vi "超标留样启动流程.vi"   [LabVIEW 2016, in "超标留样集成.lvlib" / "德润DR803M超标留样.lvlib"]
types:
  T1 = cluster{"仪器时间":timestamp, "工作状态":u16, "工作进程":u16, "采样模式":u16, "采样瓶数":dbl, "当前瓶号":dbl, "设定平行样数":dbl, "已采平行样":dbl, "设定每瓶采样次数":dbl, "已采次数":dbl, "当前瓶采样量":dbl, "瞬时流量":dbl, "累积流量":dbl, "混匀桶已采次数":dbl, "COD":dbl, "NH3N":dbl, "门状态":u16, "采样泵使能":dbl, "采样泵方向":dbl, "导流电机使能":dbl, "导流电机方向":dbl, "阀A":dbl, "阀B":dbl, "阀C":dbl, "外置泵":dbl, "预留":dbl}
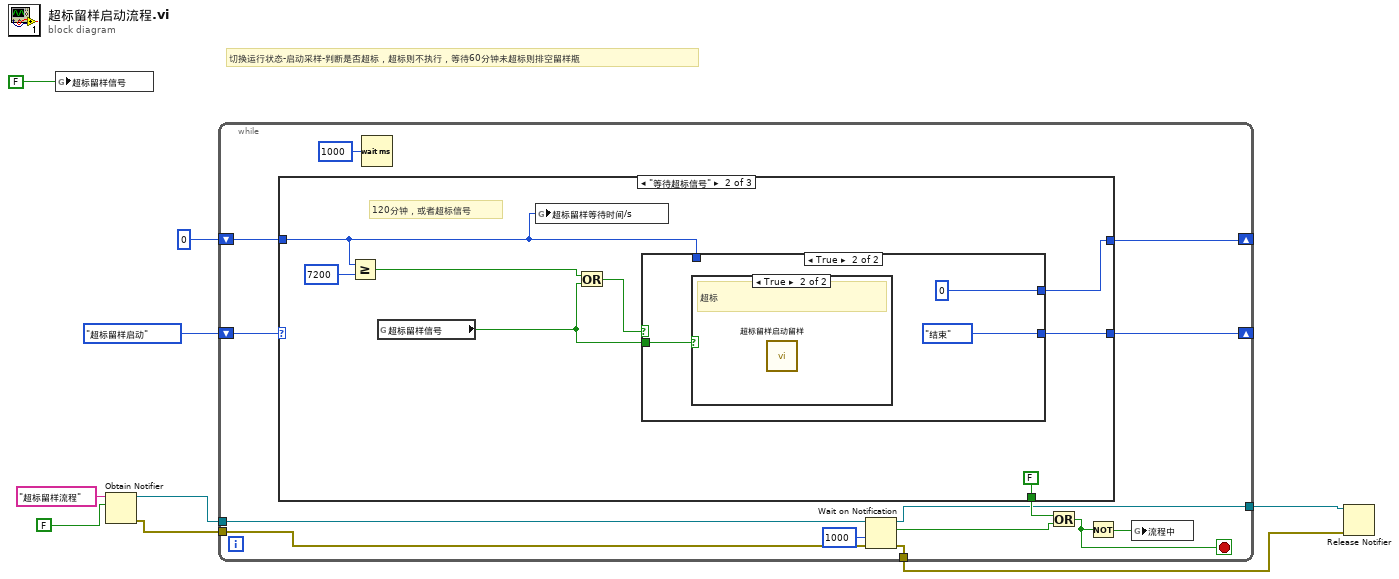
[diagram p0: block diagram]
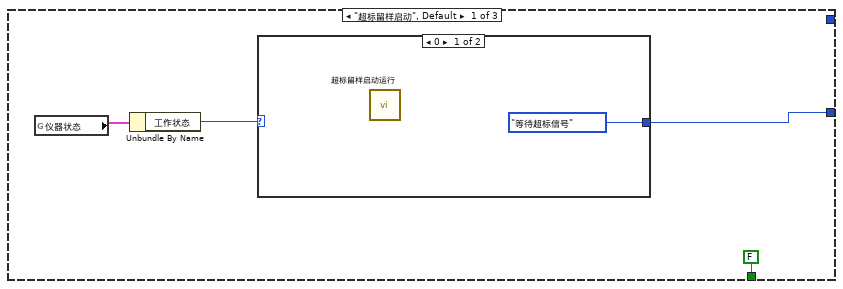
[diagram p2: hidden frame]
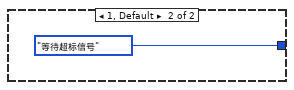
[diagram p3: hidden frame]
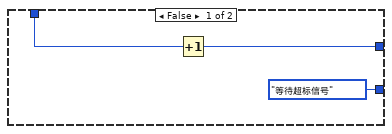
[diagram p4: hidden frame]
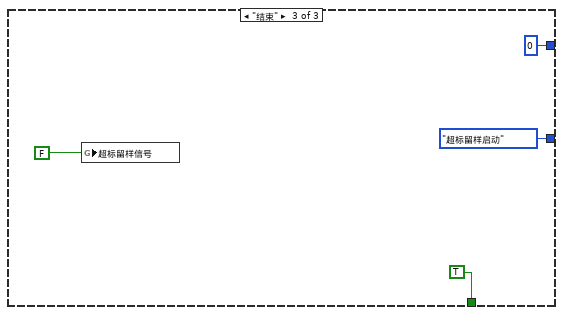
[diagram p6: hidden frame]
diagram:
  # "切换运行状态-启动采样-判断是否超标，超标则不执行，等待60分钟未超标则排空留样瓶"
  n1 = global write "超标留样全局.vi" "超标留样信号"(FALSE ("采样完成")) -> ()
  n2 = Obtain Notifier(name (unnamed)="超标留样流程" ("名称（未命名）"), notification data type=FALSE ("采样完成")) -> (notifier out=w5:refnum<notifier>, error out=w4:errorcluster)  [unwired: 2 in, 1 out]
  n3 = while {
    shift-right: [w13] -> _
    shift-left: enum16{"超标留样启动", "等待超标信号", "结束"}."超标留样启动" -> [w23]
    shift-right: [w20] -> _
    shift-left: 0 -> [w21]
    tunnel: w5 -> [w19]
    tunnel: w4 -> [w18]
    tunnel: [w11] -> w2
    tunnel: [w10] -> w1
    stop <- w16 stop-if-true
    n4 = case shown="\"等待超标信号\"" w23 {
      tunnel: w21 -> [_ w30 _]
      tunnel: [_ w35 0] -> w20
      tunnel: [w24 w33 enum16{"超标留样启动", "等待超标信号", "结束"}."超标留样启动"] -> w13
      tunnel: [FALSE FALSE TRUE] -> w12
      frame "超标留样启动", Default {
        n5 = global read "超标留样全局.vi" "仪器状态"() -> (w27:T1)
        n6 = Unbundle By Name(w27) -> ("工作状态"=w25:u16)
        n7 = case shown="0" w25 {
          tunnel: [enum16{"超标留样启动", "等待超标信号", "结束"}."等待超标信号" enum16{"超标留样启动", "等待超标信号", "结束"}."等待超标信号"] -> w24
          frame 0 {
            n8 = call "超标留样启动运行.vi"() -> ()  [unwired: 11 in, 1 out]
          }
          frame 1, Default {
          }
        }
      }
      frame "等待超标信号" {
        # "120分钟，或者超标信号"
        n9 = Greater Or Equal?(x=w30, y=7200) -> (x >= y?=w36:bool)
        n10 = global read "超标留样全局.vi" "超标留样信号"() -> (w32:bool)
        n11 = global write "超标留样全局.vi" "超标留样等待时间/s"(w30) -> ()
        n12 = Or(x=w36, y=w32) -> (x .or. y?=w34:bool)
        n13 = case shown="True" w34 {
          tunnel: [enum16{"超标留样启动", "等待超标信号", "结束"}."等待超标信号" enum16{"超标留样启动", "等待超标信号", "结束"}."结束"] -> w33
          tunnel: w30 -> [w40 _]
          tunnel: [w39 0] -> w35
          tunnel: w32 -> [_ w41]
          frame False {
            n14 = Increment(x=w40) -> (x+1=w39:i32)
          }
          frame True {
            n15 = case shown="True" w41 {
              frame False {
                # "超时但不超标"
              }
              frame True {
                # "超标"
                n16 = call "超标留样启动留样.vi"() -> ()  [unwired: 11 in, 1 out]
              }
            }
          }
        }
      }
      frame "结束" {
        n17 = global write "超标留样全局.vi" "超标留样信号"(FALSE ("采样完成")) -> ()
      }
    }
    n18 = Wait (ms)(milliseconds to wait=u32 1000 ("等待时间（毫秒）")) -> ()  [unwired: 1 out]
    n19 = Wait on Notification(notifier=w19, timeout in ms (-1)=1000 ("超时毫秒(-1)"), error in (no error)=w18) -> (notifier out=w11:refnum<notifier>, notification=w15:bool, error out=w10:errorcluster)  [unwired: 1 in, 1 out]
    n20 = Or(x=w12, y=w15) -> (x .or. y?=w16:bool)
    n21 = Not(x=w16) -> (.not. x?=w14:bool)
    n22 = global write "超标留样全局.vi" "流程中"(w14) -> ()
  }
  n23 = Release Notifier(notifier=w2, error in (no error)=w1) -> ()  [unwired: 1 in, 3 out]
